vi "Write cell value.vi"(8 "error in (no error)":errorcluster, 10 "cell value":string, 11 "CellValueChanged in":refnum<class "CellValueChanged.lvclass">) -> (0 "error out":errorcluster, 3 "CellValueChanged out":refnum<class "CellValueChanged.lvclass">)   [LabVIEW 2013, in "DataGrid.lvlib" / "CellValueChanged.lvclass"]
uses:
  CellValueChanged.lvclass
  CellValueChanged.lvclass/CellValueChanged.ctl
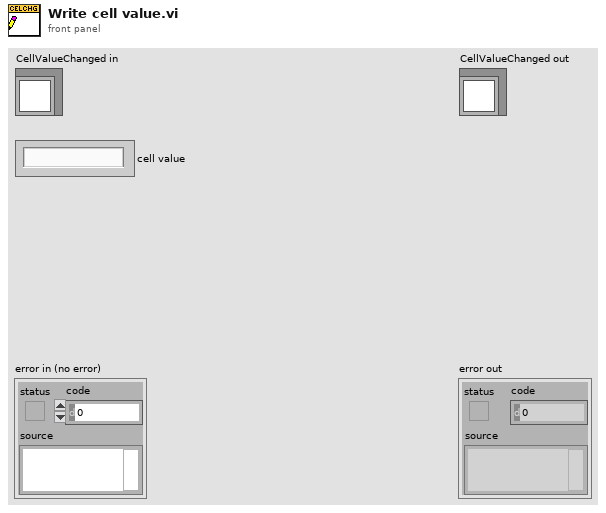
[diagram p1: front panel]
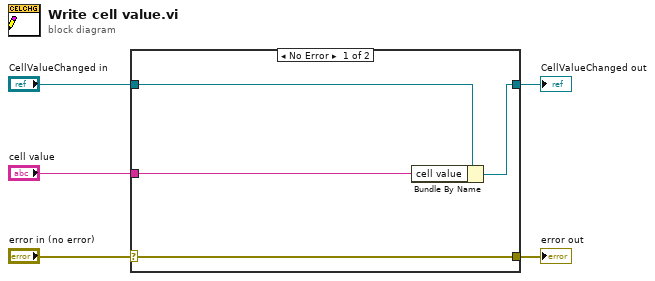
[diagram p0: block diagram]
diagram:
  n1 = case shown="No Error" "error in (no error)" {
    selector: "error in (no error)" -> [w9 w10]
    tunnel: [w9 w10] -> w4
    tunnel: [w7 w11] -> w2
    tunnel: "CellValueChanged in" -> [w8 w11]
    tunnel: "cell value" -> [w6 _]
    frame No Error {
      n2 = Bundle By Name(cluster=w8, "cell value"=w6) -> (w7:refnum<class "CellValueChanged.lvclass">)
    }
    frame Error {
    }
  }
  "error out" <- w4
  "CellValueChanged out" <- w2
